vi "Torros_Slnd.vi"(11 "Toggle?":bool) -> ()   [LabVIEW 2018]
uses:
  <vilib>/Rock Robotics/WPI/Solenoid/Deprecated/WPI_SolenoidSetBool.vi
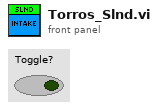
[diagram p1: front panel]
types:
  T1 = typedef "WPI_SolenoidDevRef.ctl" = cluster{"DevStatus":errorcluster, "Pneumatics Control Module":u8, "Forward Solenoid Channel":T2, "Reverse Solenoid Channel":T2}
  T2 = typedef "WPI_SolenoidChannel.ctl" = enum8{"Solenoid 0", "Solenoid 1", "Solenoid 2", "Solenoid 3", "Solenoid 4", "Solenoid 5", "Solenoid 6", "Solenoid 7", "Invalid"}
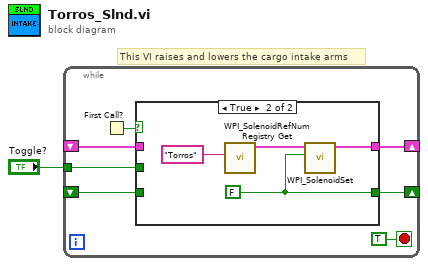
[diagram p0: block diagram]
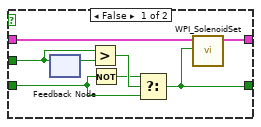
[diagram p2: hidden frame]
diagram:
  # "This VI raises and lowers the cargo intake arms"
  n1 = while {
    shift-right: [w8] -> _
    shift-left: _ -> [w6]
    tunnel: "Toggle?" -> [w7]
    shift-right: [w5] -> _
    shift-left: _ -> [w4]
    stop <- TRUE stop-if-true
    n2 = First Call?() -> (First Call?: T/F=w2:bool)
    n3 = case shown="True" w2 {
      tunnel: [w16 w18] -> w8
      tunnel: w7 -> [w14 _]
      tunnel: w6 -> [w13 _]
      tunnel: [w12 w17] -> w5
      tunnel: w4 -> [w9 _]
      frame False {
        n4 = feedback #1() -> (w15:bool)  [unwired: 1 in]
        n5 = feedback-in #1(w14) -> ()
        n6 = Greater?(x=w14, y=w15) -> (0:w11:bool)
        n7 = Not(x=w9) -> (.not. x?=w10:bool)
        n8 = Select(t=w10, s=w11, f=w9) -> (s? t:f=w12:bool)
        n9 = call-poly <vilib>:"WPI_SolenoidSet.vi"("Value"=w12, "SolenoidDevRef"=w13) -> ("SolenoidDevRef"=w16:T1)  [unwired: 8 in, 1 out]
      }
      frame True {
        w17 = FALSE
        n10 = call <vilib>:"WPI_SolenoidRefNum Registry Get.vi"("refnum name"="Torros") -> ("SolenoidDevRef"=w19:T1)  [unwired: 9 in, 1 out]
        n11 = call-poly <vilib>:"WPI_SolenoidSet.vi"("Value"=w17, "SolenoidDevRef"=w19) -> ("SolenoidDevRef"=w18:T1)  [unwired: 8 in, 1 out]
      }
    }
  }
